vi "Swing-up Control.vi"() -> ()   [LabVIEW 2019]
uses:
  <vilib>/Simulation/Scripting/Companion Diagram/SimConfigNode/SimParams.ctl
  <vilib>/Simulation/Scripting/Companion Diagram/SimConfigNode/_simSolvers.ctl
  <vilib>/Simulation/Implementation/Shared/SIMSCR Execution Mode.ctl
  <vilib>/Platform/TimedLoop/XDataNode/timing_clust.ctl
  <vilib>/Platform/TimedLoop/XDataNode/nitl_modes.ctl
  <vilib>/Platform/TimedLoop/XDataNode/wakeup.ctl
  <vilib>/Simulation/Param Hierarchy/Typedefs/SIMPH Param Control Actions.ctl
  <vilib>/Simulation/Implementation/Shared/NILVSim_ParamChanged.vi
  <vilib>/Simulation/Implementation/Shared/NILVSim_FinishedLate.vi
  <vilib>/Simulation/Implementation/Shared/NILVSIM_BeginStep.vi
  <vilib>/Simulation/Utility/Implementation/SIM Halt.vi
  <vilib>/Simulation/DataSources/Implementation/NILVSim Signal Generator.llb/SIM Signal Generator (scalar).vi
  <vilib>/Simulation/SignalDisplay/Implementation/NILVSim Time Waveform.llb/SIM Time Waveform (vector).vi
  <vilib>/Simulation/SignalDisplay/Implementation/NILVSim Time Waveform.llb/SIM Time Waveform (scalar).vi
  <vilib>/Simulation/ContinuousLinear/Implementation/NILVSim Transfer Function Direct.llb/SIM Transfer Function Direct (SISO).vi
  <vilib>/Simulation/SignalArithmetic/Implementation/NILVSim Gain.llb/SIM Gain (dot product).vi
  <vilib>/Simulation/Nonlinear/Implementation/NILVSim Saturation.llb/SIM Saturation (scalar).vi
  <vilib>/Simulation/Implementation/Shared/NILVSim_Manager.vi
  <vilib>/Utility/error.llb/Clear Errors.vi
  <vilib>/Simulation/Implementation/Shared/NILVSim_FinalizeModel.vi
  <vilib>/Simulation/Implementation/Shared/SIM Unbundle Sim Info.vi
  <vilib>/Simulation/Implementation/Shared/SIMSH Read Queue.vi
  <vilib>/Simulation/Implementation/Shared/NILVSim_Initialize.vi
  SubVIs/Encoders.vi
  <vilib>/Simulation/Utility/Implementation/NILVSim Get Time and IsAcceptedStep.vi
  SubVIs/Motor.vi
  <vilib>/Simulation/Implementation/Shared/NILVSim_GetModelError.vi
  <vilib>/Simulation/Implementation/Shared/SIM Bundle Sim Info.vi
  <vilib>/Simulation/Scripting/Companion Diagram/SimConfigNode/SimDog.xnode
  SubVIs/Swing Up Energy Control.vi
  <vilib>/Platform/TimedLoop/XDataNode/XDataNode.xnode
  <vilib>/Simulation/Implementation/XNodeFramework/SimXNode/SimX.xnode
  <vilib>/Simulation/Implementation/Shared/NI_SIM_Implementation.lvlib
  <vilib>/Platform/TimedLoop/XDataNode/XDNodeRunTimeDep.lvlib
panel:
  in  "Stop Button":bool
  in  "Signal Generator":T1={"Amplitude (deg)"=0.0, "Frequency (Hz)"=0.2} {"Frequency (Hz)" step=0.1}
  out "Pendulum Arm Angle":waveform(dbl)[](graph)=[{"t0"=timestamp(8.874 s since 1904-01-01), "dt"=1.0, "Y"=[0.0]}, {"t0"=timestamp(8.874 s since 1904-01-01), "dt"=1.0, "Y"=[4.21875]}]
  out "Pendulum Angle":waveform(dbl)(graph)={"t0"=timestamp(8.874 s since 1904-01-01), "dt"=1.0, "Y"=[0.35156250000001155]}
  out "Pendulum Energy":waveform(dbl)(graph)={"t0"=timestamp(8.874 s since 1904-01-01), "dt"=1.0, "Y"=[29.90059948688503]}
  in  "Energy Control":T2={"Er (mJ)"=30.0, "mu (m/s^2/J)"=35.0, "u_max (m/s^2)"=6.0} {"u_max (m/s^2)" min=0.0 max=10.0 step=0.5; "mu (m/s^2/J)" min=0.0 max=150.0 step=5.0; "Er (mJ)" min=0.0 max=50.0 step=5.0}
  in  "Feedback Gain":dbl[](array[numeric])=[-3.39, 41.48, -1.38, 2.94]
  out "Error":errorcluster={"status"=FALSE, "code"=-363017, "source"="ELVIS III v1.0 Write PWM.vi"}
  # "Engineering Trainer Boards"
  # "Controls Board"
  # "Swing-up Control"
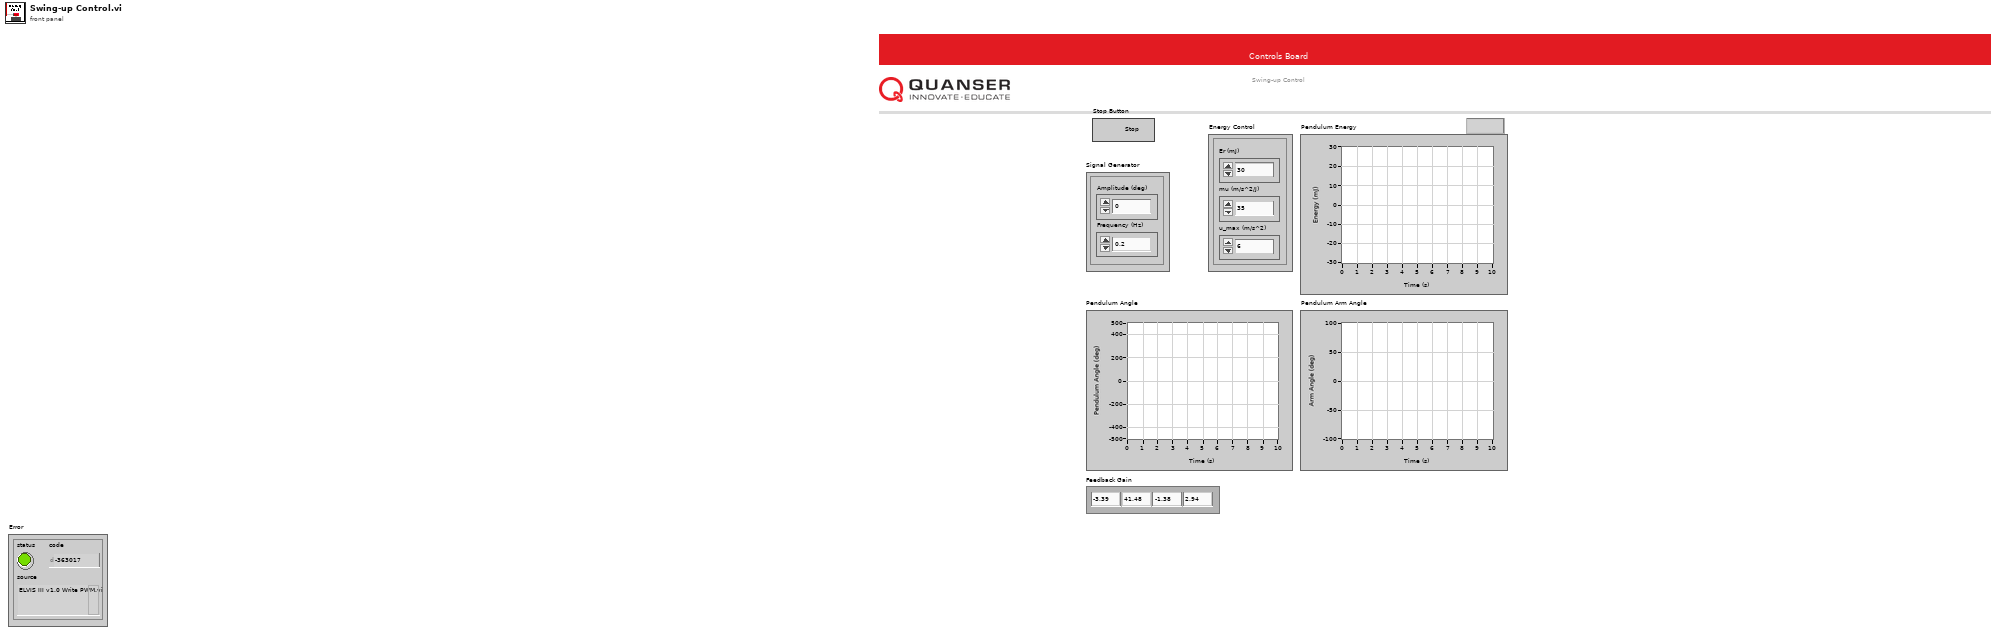
[diagram p1: front panel]
types:
  T1 = cluster{"Amplitude (deg)":dbl, "Frequency (Hz)":dbl}
  T2 = cluster{"Er (mJ)":dbl, "mu (m/s^2/J)":dbl, "u_max (m/s^2)":dbl}
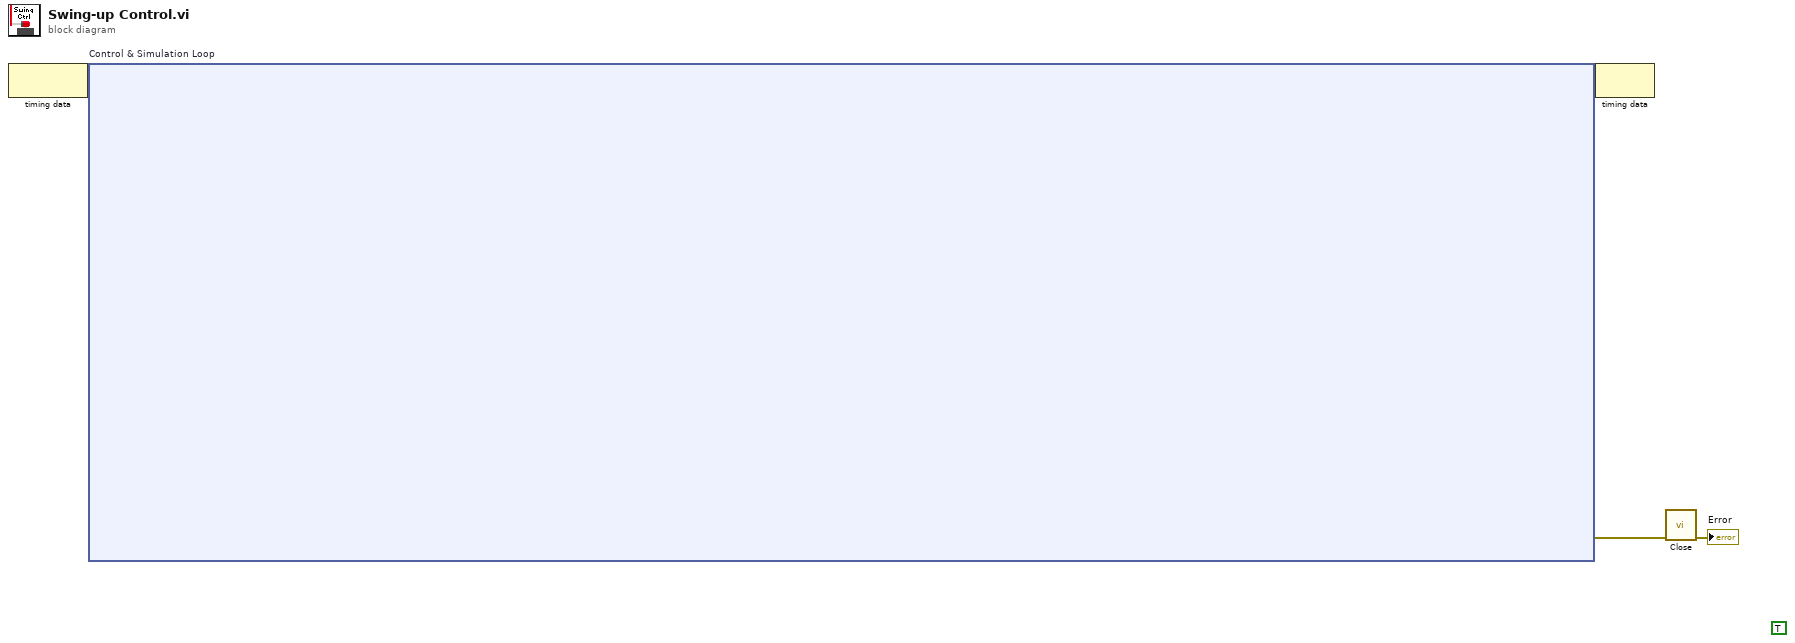
[diagram p0: block diagram]
diagram:
  (unwired) TRUE
  n1 = node-c288() -> (w4:variant)  [unwired: 1 in]
  n2 = node-c254 "Control & Simulation Loop"(w4) -> (w3:variant, w2:errorcluster)
  n3 = node-c288(w3) -> ()  [unwired: 1 out]
  n4 = call "Close.vi"("error in"=w2) -> ("error out"=→"Error":errorcluster)  [unwired: 10 in]
